vi "random personality.vi"(10 "Personalities to choose from":T1[](array[typedef])) -> (2 "Personality":T1)   [LabVIEW 2014, in "JFD_Common.lvlib"]
uses:
  JFD_Common.lvlib
  personality.ctl
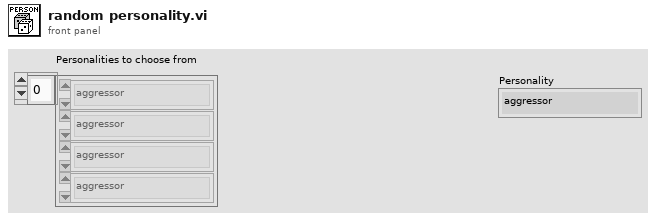
[diagram p1: front panel]
types:
  T1 = typedef "JFD_Common.lvlib/personality.ctl" = enum16{"aggressor", "replicator"}
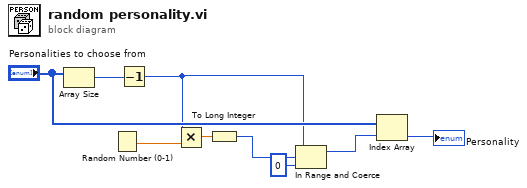
[diagram p0: block diagram]
diagram:
  n1 = Array Size(array="Personalities to choose from") -> (size(s)=w2:i32)
  n2 = Random Number (0-1)() -> (number: 0 to 1=w9:dbl)
  n3 = Decrement(x=w2) -> (x-1=w1:i32)
  n4 = Multiply(x=w1, y=w9) -> (x*y=w8:dbl)
  n5 = To Long Integer(number=w8) -> (32bit integer=w4:i32)
  n6 = In Range and Coerce(upper limit=w1, x=w4, lower limit=0) -> (coerced(x)=w3:i32)  [unwired: 1 out]
  n7 = Index Array(array="Personalities to choose from", index=w3) -> (element=→"Personality":T1)
